vi "write new child message.vi"(11 "child":refnum<class "communicator.lvclass">) -> (3 "message":refnum<class "communicator message.lvclass">)   [LabVIEW 2015, in "communicator.lvclass"]
uses:
  communicator.lvclass
  message/communicator message.lvclass
  message/communicator message.lvclass/communicator message.ctl
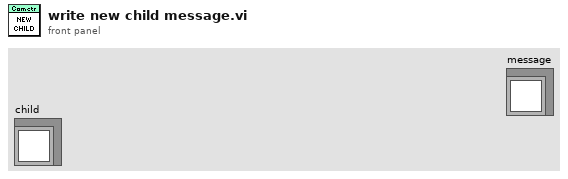
[diagram p1: front panel]
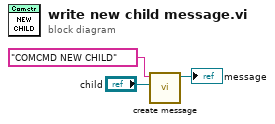
[diagram p0: block diagram]
diagram:
  n1 = call "create message.vi"("data"="child", "ID"="COMCMD NEW CHILD") -> ("message"=→"message":refnum<class "communicator message.lvclass">)  [unwired: 9 in]
